vi "DAQ.Read AI and Write AO.vi"(8 "error in (no error)":errorcluster, 11 "Instrument.DAQ in":refnum<class "Instrument.DAQ.lvclass">) -> (0 "error out":errorcluster, 3 "Instrument.DAQ out":refnum<class "Instrument.DAQ.lvclass">)   [LabVIEW 2019, in "Instrument.DAQ.lvclass"]
uses:
  Instrument.DAQ.lvclass
  Instrument.DAQ.lvclass/Instrument.DAQ.ctl
panel:
  out "Waveform Graph":waveform(dbl)[](graph)
  out "AO (ms)":u32
  out "AI (ms)":u32
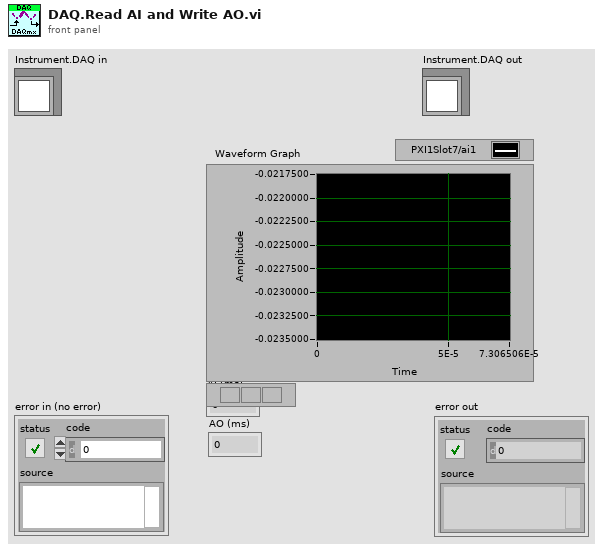
[diagram p1: front panel]
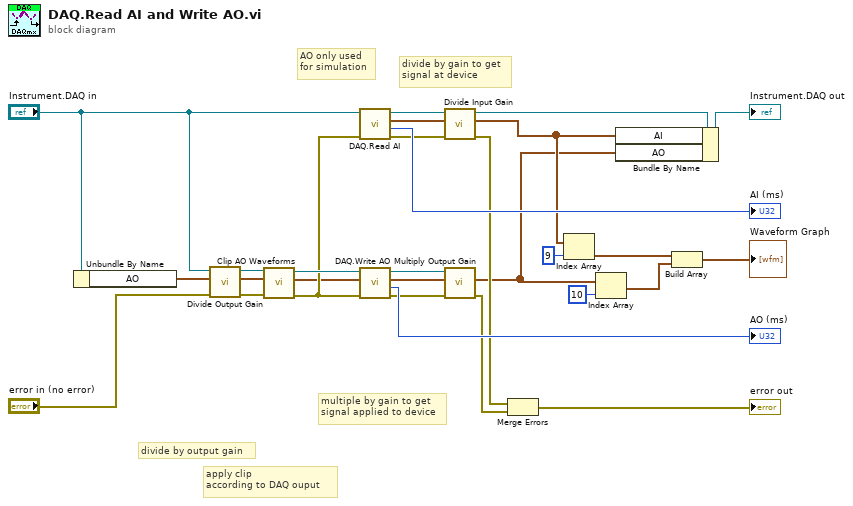
[diagram p0: block diagram]
diagram:
  # "divide by gain to get\nsignal at device"
  # "multiple by gain to get\nsignal applied to device"
  # "apply clip\naccording to DAQ ouput"
  # "divide by output gain"
  # "AO only used\nfor simulation"
  n1 = Unbundle By Name("Instrument.DAQ in") -> ("AO"=w10:waveform(dbl)[])
  n2 = call "Divide Output Gain.vi"("error in (no error)"="error in (no error)", "WFM in"=w10, "Instrument.DAQ"="Instrument.DAQ in") -> ("error out"=w25:errorcluster, "WFM out"=w27:waveform(dbl)[], "Instrument.DAQ out"=w26:refnum<class "Instrument.DAQ.lvclass">)  [unwired: 6 in]
  n3 = call "Clip AO Waveforms.vi"("error in (no error)"=w25, "AO []"=w27, "Instrument.DAQ in"=w26) -> ("error out"=w23:errorcluster, "Clipped AO []"=w12:waveform(dbl)[], "Instrument.DAQ out"=w24:refnum<class "Instrument.DAQ.lvclass">)  [unwired: 6 in]
  n4 = call "DAQ.Read AI.vi"("error in"=w23, "Instrument.DAQ in"="Instrument.DAQ in") -> ("error out"=w19:errorcluster, "AI time (ms)"=→"AI (ms)":u32, "AI []"=w21:waveform(dbl)[], "Instrument.DAQ out"=w20:refnum<class "Instrument.DAQ.lvclass">)  [unwired: 6 in]
  n5 = call "DAQ.Write AO.vi"("error in (no error)"=w23, "AO []"=w12, "Instrument.DAQ in"=w24) -> ("error out"=w18:errorcluster, "AO time (ms)"=→"AO (ms)":u32, "AO out []"=w16:waveform(dbl)[], "Instrument.DAQ out"=w22:refnum<class "Instrument.DAQ.lvclass">)  [unwired: 5 in]
  n6 = call "Divide Input Gain.vi"("error in (no error)"=w19, "WFM in"=w21, "Instrument.DAQ"=w20) -> ("error out"=w14:errorcluster, "WFM out"=w7:waveform(dbl)[], "Instrument.DAQ out"=w9:refnum<class "Instrument.DAQ.lvclass">)  [unwired: 6 in]
  n7 = call "Multiply Output Gain.vi"("error in (no error)"=w18, "WFM in"=w16, "Instrument.DAQ"=w22) -> ("error out"=w13:errorcluster, "WFM out"=w6:waveform(dbl)[])  [unwired: 6 in, 1 out]
  n8 = Merge Errors(w14, w13) -> (→"error out":errorcluster)
  n9 = Index Array(array=w7, index=9) -> (element=w3:waveform(dbl))
  n10 = Index Array(array=w6, index=10) -> (element=w2:waveform(dbl))
  n11 = Bundle By Name(cluster=w9, "AI"=w7, "AO"=w6) -> (→"Instrument.DAQ out":refnum<class "Instrument.DAQ.lvclass">)
  n12 = Build Array(w3, w2) -> (→"Waveform Graph":waveform(dbl)[])
